vi "SetTrafficLightRef.vi"(0 "object in":refnum<class "RedState.lvclass">, 1 "TrafficLightRef":refnum<class "TrafficLight.lvclass">, 5 "Error In":errorcluster) -> (14 "object out":refnum<class "RedState.lvclass">, 19 "Error Out":errorcluster)   [LabVIEW 2024, in "RedState.lvclass"]
uses:
  RedState.lvclass
  TrafficLight_class/TrafficLight.lvclass
  RedState.lvclass/RedState.ctl
panel:
  # "Connector Pane"
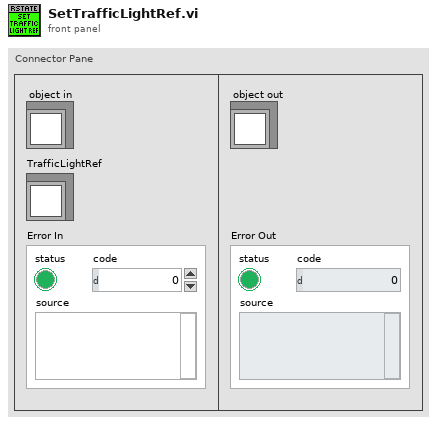
[diagram p1: front panel]
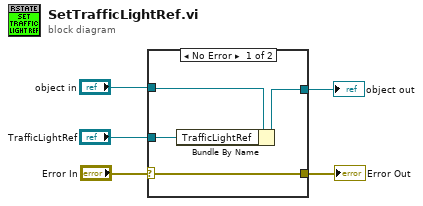
[diagram p0: block diagram]
diagram:
  n1 = case shown="No Error" "Error In" {
    selector: "Error In" -> [w8 w11]
    tunnel: [w8 w11] -> w4
    tunnel: [w6 w10] -> w2
    tunnel: "object in" -> [w7 w10]
    tunnel: "TrafficLightRef" -> [w9 _]
    frame No Error {
      n2 = Bundle By Name(cluster=w7, "TrafficLightRef"=w9) -> (w6:refnum<class "RedState.lvclass">)
    }
    frame Error {
    }
  }
  "Error Out" <- w4
  "object out" <- w2
